vi "CicloWhile.vi"() -> ()   [LabVIEW 2021]
panel:
  out "Array":dbl[](array[numeric])
  out "Numeric":dbl
  out "Waveform Chart":dbl(graph)
  in  "Slide":u32(slide) scale=1.0..2000.0
  in  "stop":bool
  out "Numeric":i32
  # "Mendoza Meza Manuel Everardo"
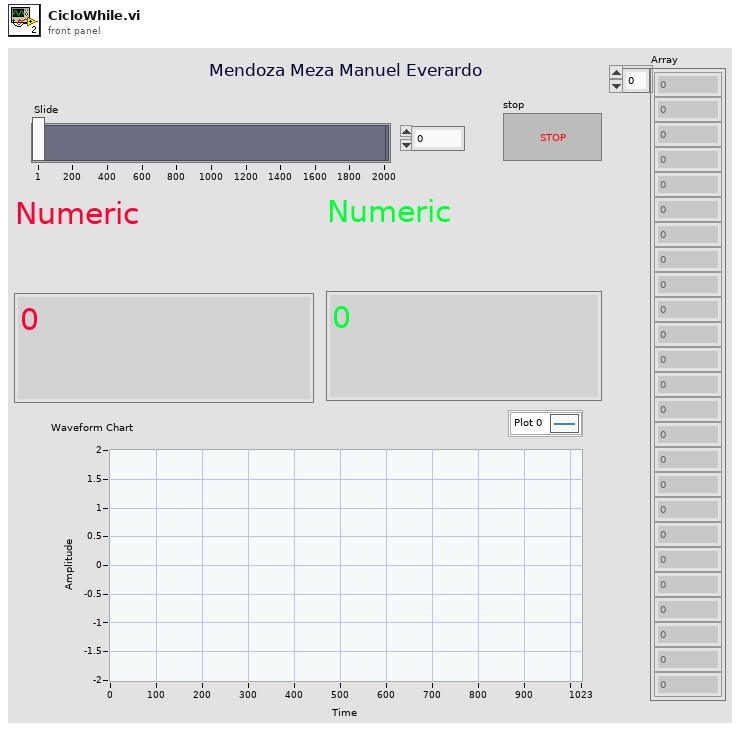
[diagram p1: front panel]
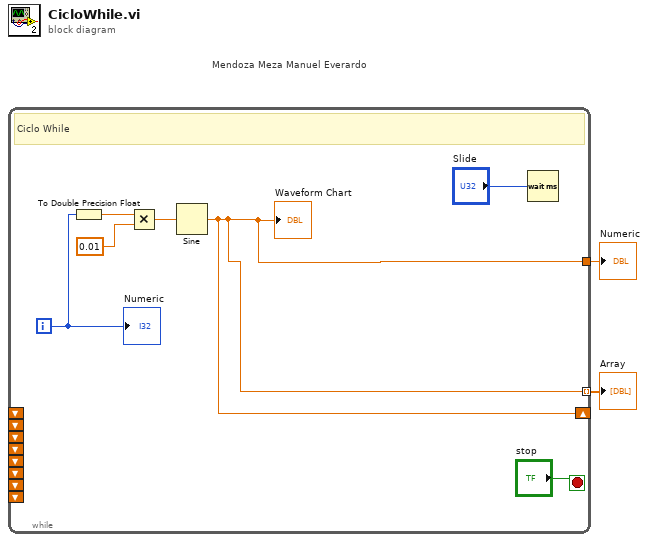
[diagram p0: block diagram]
diagram:
  # "Mendoza Meza Manuel Everardo"
  n1 = while {
    tunnel: [w3] -> w2
    tunnel: [w3] -> w1 mode=indexing
    shift-right: [w3] -> _
    shift-left: _ -> [_]
    shift-left: _ -> [_]
    shift-left: _ -> [_]
    shift-left: _ -> [_]
    shift-left: _ -> [_]
    shift-left: _ -> [_]
    shift-left: _ -> [_]
    shift-left: _ -> [_]
    i -> [w6]
    stop <- "stop" stop-if-true
    # "Ciclo While"
    n2 = To Double Precision Float(number=w6) -> (double precision float=w7:dbl)
    n3 = Multiply(x=w7, y=0.01) -> (x*y=w4:dbl)
    n4 = Sine(x=w4) -> (sin(x)=w3:dbl)
    "Waveform Chart" <- w3
    n5 = Wait (ms)(milliseconds to wait="Slide") -> ()  [unwired: 1 out]
    "Numeric" <- w6
  }
  "Numeric" <- w2
  "Array" <- w1
